vi "DHE_GetDBS.vi"() -> (7 "DHE_DBSRef":T1)   [LabVIEW 2016]
uses:
  DBSHAND/private/vis/DatabaseHand_RefNum.ctl
  private/vis/DHE_GBLDriverVariables.vi
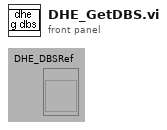
[diagram p1: front panel]
types:
  T1 = typedef "DatabaseHand_RefNum.ctl" = refnum<vi>
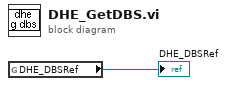
[diagram p0: block diagram]
diagram:
  n1 = global read "DHE_GBLDriverVariables.vi" "DHE_DBSRef"() -> (→"DHE_DBSRef":T1)
